vi "CABLE_SetCuff_Shank.vi"(9 "ExtraWeight":dbl, 10 "Distance To Knee":dbl=0.15, 11 "Shank Length":dbl=0.42 format="%#_13g") -> (3 "Shank Cuff":T1={"BodyID"=0, "CoM(CuffCS)"={"Coord4"=[0.0, 0.0, 0.0, 1.0], "ID"=0}, "Mass(kg)"=0.0, "CablePts(CuffCS)"=[], "Cuff->Body"=[[1.0, 0.0, 0.0, 0.0], [0.0, 1.0, 0.0, 0.0], [0.0, 0.0, 1.0, 0.0], [0.0, 0.0, 0.0, 1.0]]})   [LabVIEW 2016, in "CAlex2.lvclass"]
uses:
  CAlex2.lvclass
  SerialChain-Cable/TypeDef/Cuff.ctl
  SerialChain/TypeDef/PointOnBody.ctl
  <vilib>/Analysis/Matrix/Datatypes/RealMatrix.ctl
  SerialChain/TypeDef/xyzO.ctl
  <vilib>/Analysis/Matrix/NI_Matrix.lvlib
  SerialChain/SerialChain.lvclass
  SerialChain-Cable/SerialChain-Cable.lvclass
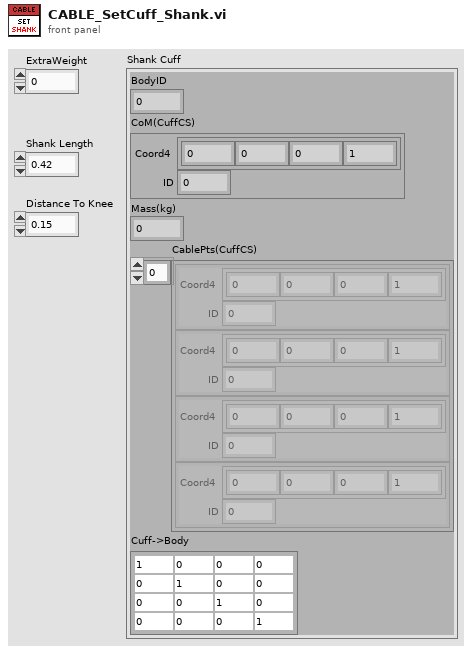
[diagram p1: front panel]
types:
  T1 = typedef "SerialChain-Cable.lvclass/Cuff.ctl" = cluster{"BodyID":i32, "CoM(CuffCS)":T2, "Mass(kg)":dbl, "CablePts(CuffCS)":T2[], "Cuff->Body":T3}
  T2 = typedef "SerialChain.lvclass/PointOnBody.ctl" = cluster{"Coord4":dbl[], "ID":i32}
  T3 = typedef "NI_Matrix.lvlib/RealMatrix.ctl" = dbl[][]
  T4 = typedef "SerialChain.lvclass/xyzO.ctl" = enum16{"X", "Y", "Z", "O"}
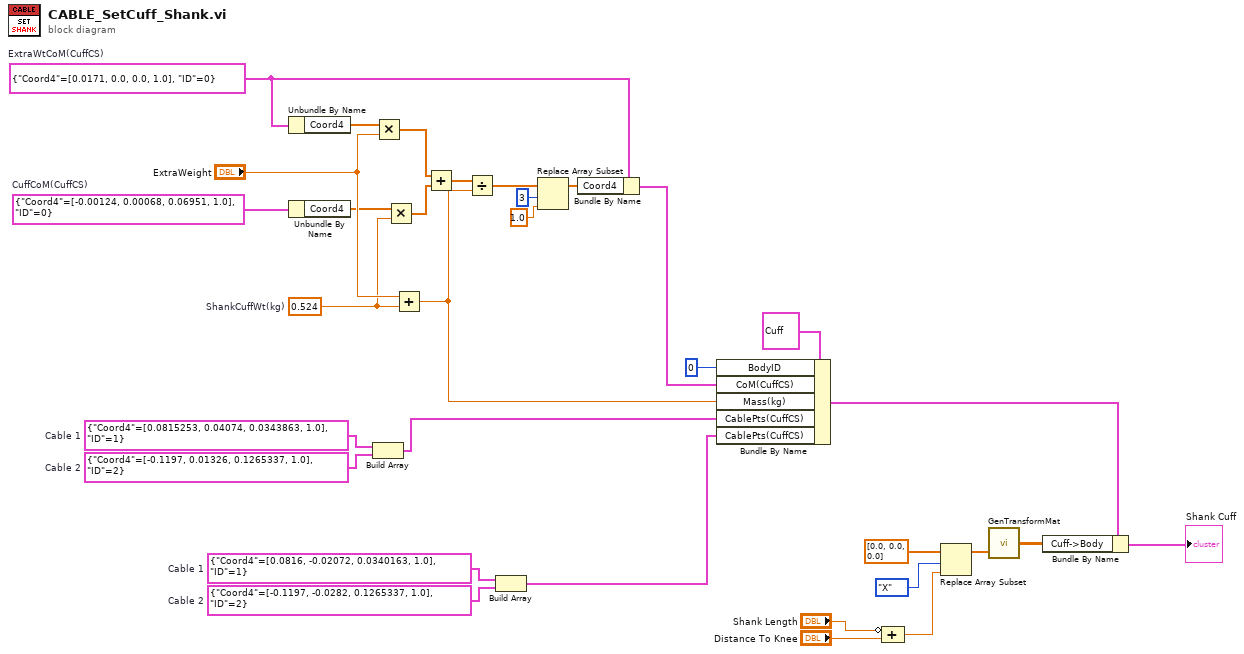
[diagram p0: block diagram]
diagram:
  w2 = T2 {"Coord4"=[-0.1197, 0.01326, 0.1265337, 1.0], "ID"=2}  # Cable 2
  w3 = T2 {"Coord4"=[0.0815253, 0.04074, 0.0343863, 1.0], "ID"=1}  # Cable 1
  w22 = T2 {"Coord4"=[0.0171, 0.0, 0.0, 1.0], "ID"=0}  # ExtraWtCoM(CuffCS)
  w29 = T2 {"Coord4"=[-0.1197, -0.0282, 0.1265337, 1.0], "ID"=2}  # Cable 2
  w30 = T2 {"Coord4"=[0.0816, -0.02072, 0.0340163, 1.0], "ID"=1}  # Cable 1
  w14 = 0.524  # ShankCuffWt(kg)
  w16 = T2 {"Coord4"=[-0.00124, 0.00068, 0.06951, 1.0], "ID"=0}  # CuffCoM(CuffCS)
  n1 = Unbundle By Name(w22) -> ("Coord4"=w28:dbl[])
  n2 = Unbundle By Name(w16) -> ("Coord4"=w26:dbl[])
  n3 = Build Array(w3, w2) -> (w1:T2[])
  n4 = Multiply(x=w28, y="ExtraWeight") -> (x*y=w25:dbl[])
  n5 = Multiply(x=w26, y=w14) -> (x*y=w24:dbl[])
  n6 = Add(x="ExtraWeight", y=w14) -> (x+y=w15:dbl)
  n7 = Add(x=w25, y=w24) -> (x+y=w23:dbl[])
  n8 = Divide(x=w23, y=w15) -> (x/y=w21:dbl[])
  n9 = Build Array(w30, w29) -> (w4:T2[])
  n10 = Replace Array Subset(array=w21, new element=1.0 ("new element/subarray"), index=3) -> (w20:dbl[])
  n11 = Bundle By Name(cluster=w22, "Coord4"=w20) -> (w17:T2)
  n12 = Bundle By Name(cluster=T1 {"BodyID"=0, "CoM(CuffCS)"={"Coord4"=[0.0, 0.0, 0.0, 1.0], "ID"=0}, "Mass(kg)"=0.0, "CablePts(CuffCS)"=[], "Cuff->Body"=[[1.0, 0.0, 0.0, 0.0], [0.0, 1.0, 0.0, 0.0], [0.0, 0.0, 1.0, 0.0], [0.0, 0.0, 0.0, 1.0]]} ("Cuff Design"), "BodyID"=0, "CoM(CuffCS)"=w17, "Mass(kg)"=w15, "CablePts(CuffCS)"=w1, "CablePts(CuffCS)"=w4) -> (w13:T1)
  n13 = Compound Arithmetic op=ADD(invert "Shank Length", "Distance To Knee") -> (w5:dbl)
  n14 = Replace Array Subset(array=dbl[] [0.0, 0.0, 0.0], new element=w5, index=xyzO."X" ("XYZ")) -> (w10:dbl[])
  n15 = call "GenTransformMat.vi"("Translate 3Vector"=w10) -> ("Transformation Matrix"=w8:T3)  [unwired: 1 in]
  n16 = Bundle By Name(cluster=w13, "Cuff->Body"=w8) -> (→"Shank Cuff":T1)
